vi "AcquireSpatialCam.vi"(8 "error in (no error)":errorcluster, 11 "FROG in":refnum<class "FROG.lvclass">) -> (0 "error out":errorcluster, 3 "FROG out":refnum<class "FROG.lvclass">)   [LabVIEW 2020, in "FROG.lvclass"]
uses:
  FROG.lvclass
  FROG.lvclass/FROG.ctl
  Point Grey Camera/GUIcompressionCluster.ctl
  shared/OnOffTypeDef.ctl
  shared/CompressAndUpdate(Poly)/CompressAndUpdate(IMAQ Image).vi
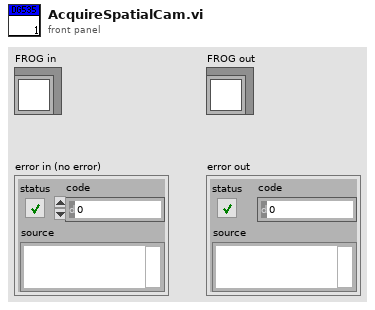
[diagram p1: front panel]
types:
  T1 = typedef "IMAQ Image.ctl" = refnum<image>
  T2 = typedef "GUIcompressionCluster.ctl" = cluster{"GUI8bit":T3, "GUICompression":T3, "CompressionQuality":i32}
  T3 = typedef "OnOffTypeDef.ctl" = enum16{"off", "on"}
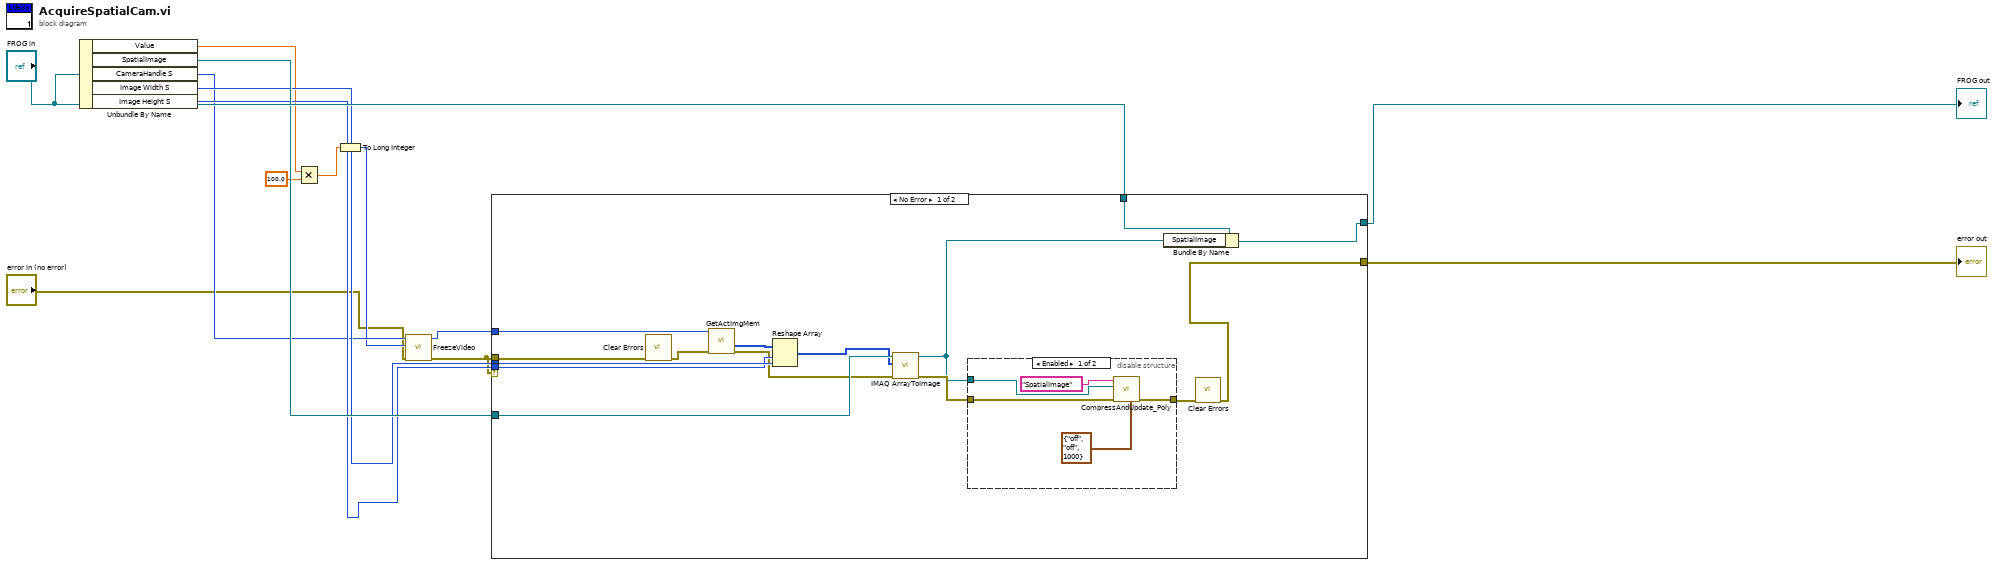
[diagram p0: block diagram]
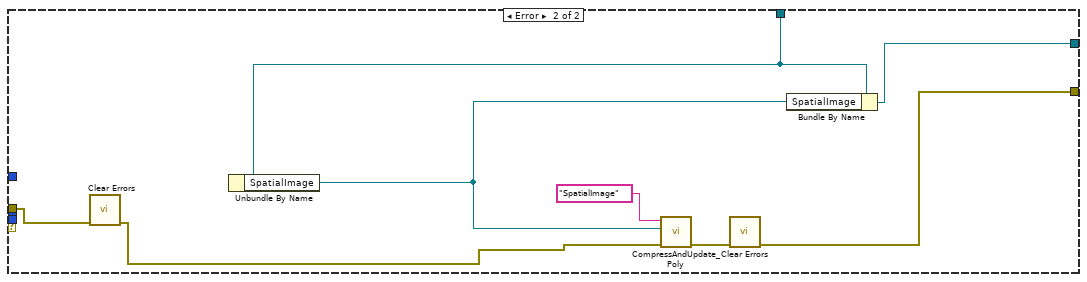
[diagram p3: hidden frame]
diagram:
  n1 = Unbundle By Name ("pressure read")("FROG in") -> ("Value"=w7:dbl, "SpatialImage"=w13:T1, "CameraHandle S"=w10:u32, "Image Width S"=w11:i32, "Image Height S"=w12:i32)
  n2 = Multiply(x=w7, y=100.0) -> (x*y=w6:dbl)
  n3 = To Long Integer(number=w6) -> (32bit integer=w9:i32)
  n4 = call "FreezeVideo.vi"("error in"="error in (no error)", "Wait"=w9, "Camera Handle In"=w10) -> ("error out"=w4:errorcluster, "Camera Handle Out"=w3:u32)  [unwired: 7 out]
  n5 = case shown="No Error" w4 {
    tunnel: w13 -> [w29 _]
    tunnel: w11 -> [w28 _]
    tunnel: w12 -> [w27 _]
    tunnel: [w26 w40] -> w2
    tunnel: w4 -> [w23 w43]
    tunnel: w3 -> [w22 _]
    tunnel: "FROG in" -> [w17 w37]
    tunnel: [w16 w39] -> w5
    frame No Error {
      n6 = call <vilib>:"Clear Errors.vi"("error in (no error)"=w23) -> ("error out"=w20:errorcluster)  [unwired: 5 in, 1 out]
      n7 = call "GetActImgMem.vi"("error in"=w20, "Camera Handle In"=w22) -> ("error out"=w25:errorcluster, "Image Memory Out"=w21:u8[])  [unwired: 8 out]
      n8 = Reshape Array(w21, w27, w28) -> (w15:u8[][])
      n9 = call "IMAQ ArrayToImage"("error in (no error)"=w25, "Image Pixels (U8)"=w15, "Image"=w29) -> ("error out"=w24:errorcluster, "Image Out"=w18:T1)  [unwired: 7 in]
      n10 = disable-structure shown="Enabled" {
        disable-tunnel: w24 -> [w33 w35]
        disable-tunnel: [w32 w35] -> w19
        disable-tunnel: w18 -> [w31 _]
        frame Enabled {
          n11 = call-poly "CompressAndUpdate_Poly.vi"("GUICompression"=T2 {"GUI8bit"=enum."off", "GUICompression"=enum."off", "CompressionQuality"=1000}, "error in"=w33, "IMAQ Image"=w31, "command or variable name"="SpatialImage") -> ("error out"=w32:errorcluster)  [unwired: 7 in]
        }
        frame Disabled {
        }
      }
      n12 = Bundle By Name(cluster=w17, "SpatialImage"=w18) -> (w16:refnum<class "FROG.lvclass">)
      n13 = call <vilib>:"Clear Errors.vi"("error in (no error)"=w19) -> ("error out"=w26:errorcluster)  [unwired: 5 in, 1 out]
    }
    frame Error {
      n14 = call <vilib>:"Clear Errors.vi"("error in (no error)"=w43) -> ("error out"=w36:errorcluster)  [unwired: 5 in, 1 out]
      n15 = Unbundle By Name(w37) -> ("SpatialImage"=w38:T1)
      n16 = call-poly "CompressAndUpdate_Poly.vi"("error in"=w36, "IMAQ Image"=w38, "command or variable name"="SpatialImage") -> ("error out"=w42:errorcluster)  [unwired: 8 in]
      n17 = call <vilib>:"Clear Errors.vi"("error in (no error)"=w42) -> ("error out"=w40:errorcluster)  [unwired: 5 in, 1 out]
      n18 = Bundle By Name(cluster=w37, "SpatialImage"=w38) -> (w39:refnum<class "FROG.lvclass">)
    }
  }
  "FROG out" <- w5
  "error out" <- w2
